vi "Main_GOOP4_CreateObjects_Open_GDS.vi"() -> ()   [LabVIEW 2016]
doc: "This is the main VI for the Project \"GOOP4_CreateObjects_Open_GDS.lvproj\""
uses:
  GOOP4_Sub_class/GOOP4_Sub.lvclass
  GOOP4_Base_class/GOOP4_Base.lvclass
panel:
  out "Sub Str":string
  out "Sub error out":errorcluster
  out "Base error out":errorcluster
  out "Sub i 1":i32
  out "Sub i 2":i32
  out "Base i 2":i32
  out "Base i 1":i32
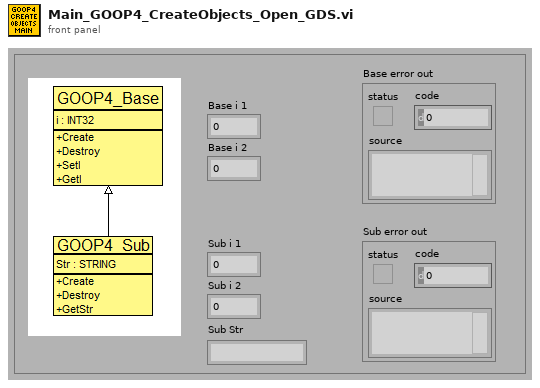
[diagram p1: front panel]
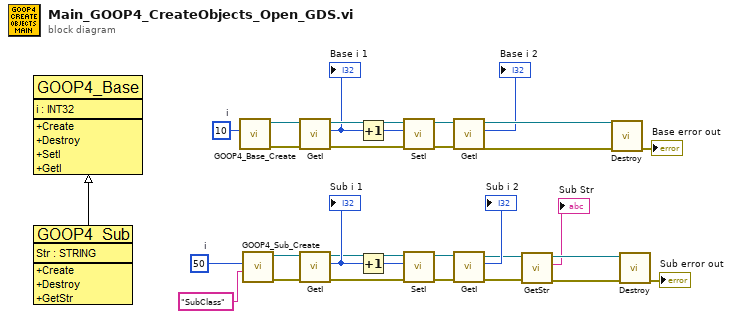
[diagram p0: block diagram]
diagram:
  w18 = 50  # i
  w26 = 10  # i
  n1 = call "GOOP4_Base_Create.vi"("i"=w26) -> ("error out"=w24:errorcluster, "reference out"=w25:refnum<class "GOOP4_Base.lvclass">)  [unwired: 9 in]
  n2 = call "GOOP4_Sub_Create.vi"("Str"="SubClass", "i"=w18) -> ("error out"=w9:errorcluster, "reference out"=w8:refnum<class "GOOP4_Sub.lvclass">)  [unwired: 8 in]
  n3 = call-dynamic "GetI.vi"("error in (no error)"=w24, "reference in"=w25) -> ("error out"=w22:errorcluster, "i"=w21:i32, "reference out"=w23:refnum<class "GOOP4_Base.lvclass">)  [unwired: 7 in]
  "Base i 1" <- w21
  n4 = call-dynamic "GetI.vi"("error in (no error)"=w9, "reference in"=w8) -> ("error out"=w13:errorcluster, "i"=w14:i32, "reference out"=w12:refnum<class "GOOP4_Sub.lvclass">)  [unwired: 7 in]
  "Sub i 1" <- w14
  n5 = Increment(x=w21) -> (x+1=w20:i32)
  n6 = Increment(x=w14) -> (x+1=w15:i32)
  n7 = call-dynamic "SetI.vi"("error in (no error)"=w22, "i"=w20, "reference in"=w23) -> ("error out"=w30:errorcluster, "reference out"=w29:refnum<class "GOOP4_Base.lvclass">)  [unwired: 7 in]
  n8 = call-dynamic "SetI.vi"("error in (no error)"=w13, "i"=w15, "reference in"=w12) -> ("error out"=w10:errorcluster, "reference out"=w11:refnum<class "GOOP4_Sub.lvclass">)  [unwired: 7 in]
  n9 = call-dynamic "GetI.vi"("error in (no error)"=w30, "reference in"=w29) -> ("error out"=w27:errorcluster, "i"=→"Base i 2":i32, "reference out"=w28:refnum<class "GOOP4_Base.lvclass">)  [unwired: 7 in]
  n10 = call-dynamic "GetI.vi"("error in (no error)"=w10, "reference in"=w11) -> ("error out"=w6:errorcluster, "i"=→"Sub i 2":i32, "reference out"=w7:refnum<class "GOOP4_Sub.lvclass">)  [unwired: 7 in]
  n11 = call-dynamic "GetStr.vi"("error in (no error)"=w6, "reference in"=w7) -> ("error out"=w4:errorcluster, "Str"=→"Sub Str":string, "reference in"=w5:refnum<class "GOOP4_Sub.lvclass">)  [unwired: 7 in]
  n12 = call-dynamic "Destroy.vi"("error in (no error)"=w27, "reference in"=w28) -> ("error out"=→"Base error out":errorcluster)  [unwired: 8 in, 1 out]
  n13 = call-dynamic "Destroy.vi"("error in (no error)"=w4, "reference in"=w5) -> ("error out"=→"Sub error out":errorcluster)  [unwired: 8 in, 1 out]
